vi "Test_API_AddSink_NoError.vi"(8 "error in (no error)":errorcluster, 11 "TestCase in":refnum<class "TestComposedLog.lvclass">) -> (0 "error out":errorcluster, 3 "TestCase out":refnum<class "TestComposedLog.lvclass">)   [LabVIEW 2017, in "TestComposedLog.lvclass"]
uses:
  TestComposedLog.lvclass
  Source/Composed Log/LoggerReference/LoggerReference.lvclass/LoggerReference.ctl
  82c09fb5-0290-453f-b865-6db4838cb6ea.vi
  74fec1c9-1b6c-42af-890e-a8b9e81c1d81.vi
  82c09fb5-0290-453f-b865-6db4838cb6ea.vi/9270b367-be30-491e-903f-1ba32711599c.vi
  74fec1c9-1b6c-42af-890e-a8b9e81c1d81.vi/83cd3f20-fe6a-4f66-9a27-0edc0c7a95eb.vi
  Source/Composed Log/LoggerReference/Return Aggregate Queues.vi
  Source/Composed Log/LoggerReference/Add Aggregate Log.vi
  82c09fb5-0290-453f-b865-6db4838cb6ea.vi/9270b367-be30-491e-903f-1ba32711599c.vi/1bd02de7-20ce-45d4-999e-e20f6b4fab2d.vi
  Source/Composed Log/LoggerReference/Send Add Sink.vi
  Source/LVQueue Sink/LVQueue Sink.lvclass
  C:/CS/Internal/LabVIEW/Logger/Source/Composed Log/Log Sink/Log Sink.lvclass
  Source/Composed Log/Application Logger/Launch Worker Loop.vi
  Source/Composed Log/LoggerReference/Initialize Logger Instance.vi
  Source/Composed Log/Singleton Event Log/Logger Queue FGV.vi
  Source/Composed Log/IErrorFormat/IErrorFormat.lvclass
  Source/Composed Log/LoggerReference/LoggerReference.lvclass
  Source/Composed Log/Log Sink/Log Sink.lvclass
  <vilib>/addons/_JKI Toolkits/VI Tester/TestCase.llb/TestCase.lvclass
  Source/Composed Log/Singleton Event Log/Singleton Event Log.lvlib
  C:/Program Files (x86)/National Instruments/LabVIEW 2017/vi.lib/addons/_JKI Toolkits/VI Tester/TestCase.llb/TestCase.lvclass
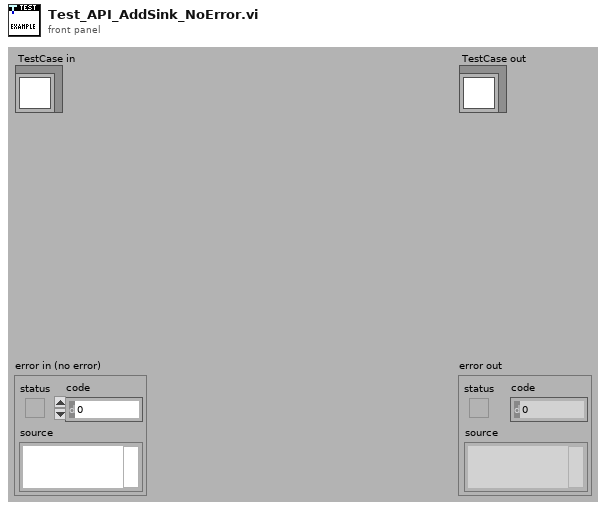
[diagram p1: front panel]
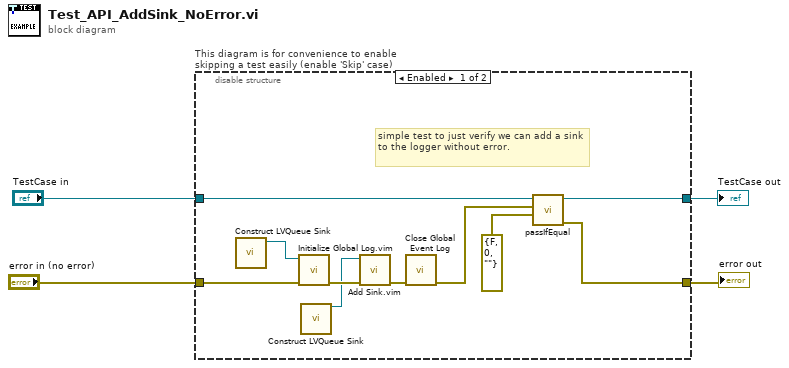
[diagram p0: block diagram]
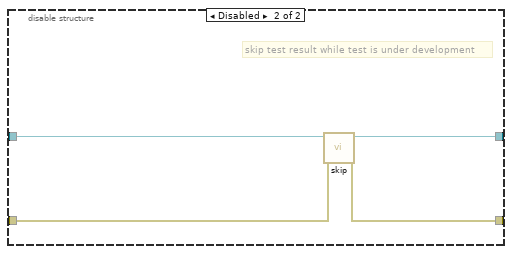
[diagram p2: hidden frame]
diagram:
  n1 = disable-structure "This diagram is for convenience to enable skipping a test easily (enable 'Skip' case)" shown="Enabled" {
    disable-tunnel: "TestCase in" -> [w13 w18]
    disable-tunnel: [w14 w16] -> w1
    disable-tunnel: [w10 w17] -> w3
    disable-tunnel: "error in (no error)" -> [w9 w15]
    frame Enabled {
      # "simple test to just verify we can add a sink to the logger without error."
      n2 = call "Construct LVQueue Sink.vi"() -> ("LVQueue Sink out"=w5:refnum<class "LVQueue Sink.lvclass">)  [unwired: 10 in, 1 out]
      n3 = call "Initialize Global Log.vim"("error in (no error)"=w9, "Log Sink(s)"=w5) -> ("error out"=w8:errorcluster)  [unwired: 8 in, 1 out]
      n4 = call "Construct LVQueue Sink.vi"() -> ("LVQueue Sink out"=w6:refnum<class "LVQueue Sink.lvclass">)  [unwired: 10 in, 1 out]
      n5 = call "Add Sink.vim"("error in (no error)"=w8, "Log Sink(s)"=w6) -> ("error out"=w7:errorcluster)  [unwired: 8 in, 1 out]
      n6 = call "Close Global Event Log.vi"("error in (no error)"=w7) -> ("error out"=w11:errorcluster)  [unwired: 10 in]
      n7 = call-dynamic "passIfEqual.vi"("y"=errorcluster {"status"=FALSE, "code"=0, "source"=""} ("error out"), "x"=w11, "TestCase in"=w13) -> ("error out"=w10:errorcluster, "TestCase out"=w14:refnum<class "TestComposedLog.lvclass">)  [unwired: 7 in]
    }
    frame Disabled {
      # "skip test result while test is under development"
      n8 = call <vilib>:"skip.vi"("error in (no error)"=w15, "TestCase in"=w18) -> ("error out"=w17:errorcluster, "TestCase out"=w16:refnum<class "TestComposedLog.lvclass">)  [unwired: 8 in]
    }
  }
  "error out" <- w3
  "TestCase out" <- w1
